vi "hardware_configurator.vi"() -> ()   [LabVIEW 2018]
doc: "MeasGUI - Measurement Graphics User Interface\nCopyright (c) 2018 Frans Korhonen\n\nMeasGUI was originally developed at Institute for Atmospheric \nand Earth System Research / Physics, Faculty of Science, \nUniversity of Helsinki, Finland\n\nAssistance, experience and feedback from following persons have been \ncritical in development of MeasGUI: Michel Attoui, Juha Kangasluoma, \nLauri Ahonen, Ella Häkkinen, Markku Kulmala and Tuukka Petäjä.\n\nThis file is part of MeasGUI.\n\nThis Source Code Form is subject to the terms of the Mozilla Public\nLicense, v. 2.0. If a copy of the MPL was not distributed with this\nfile, You can obtain one at http://mozilla.org/MPL/2.0/."
panel:
  in  "file cluster":T1={"open program folder"=FALSE, "Load"=FALSE, "Save"=FALSE, "Saved Configuration"="default", "output filename"="hardware.ini", "output"=FALSE}
  out "program path":path=path "C:/Users/fkorhone/projects/dmps_gui"
  out "saved controls":string[](array[string])=["NI measurement devices", "Serial ports"]
  in  "Tab Control":T2(tab)
  in  "NI measurement devices":T3(array[cluster])=[{"channel name"="NI1", "Device identifier"="Dev1", "analog outputs"=[{"channel name"="AO0", "terminal"="AO0"}, {"channel name"="AO1", "terminal"="AO1"}], "counter inputs"=[{"channel name"="counter", "resource"="ctr1", "terminal"="PFI0"}], "analog inputs"=[{"terminal"="AI0", "channel name"="AI0", "input terminal conf"="RSE", "signal min"=-10.0, "signal max"=10.0}, {"terminal"="AI1", "channel name"="AI1", "input terminal conf"="RSE", "signal min"=-10.0, "signal max"=10.0}], "pwm outputs"=[], "update period"=0.0, "sample rate"=0, "n average"=0}] {"update period" format="%.2f"}
  in  "Serial ports":T4(array[cluster])=[{"channel name"="serial1", "com port"="com10"}, {"channel name"="serial2", "com port"="com11"}, {"channel name"="serial3", "com port"="com12"}, {"channel name"="serial4", "com port"="com13"}]
  out "configuration":string="#CAUTION: Automatically generated file. Handmade modifications may be lost.\n\n#NI input device configuration:\ncreate niaidev NI1\ncreate timer NI1_period\nconf NI1_period 0.1\nconf NI1 Dev1 1000 10\n\n#Analog inputs:\ncreate niai AI0\nconf AI0 NI1 AI0 RSE -10.000000 10.000000\ncreate niai AI1\nconf AI1 NI1 AI1 RSE -10.000000 10.000000\n\nlink NI1_period NI1\n\n#Counter inputs:\ncreate nicounter counter\nsetup counter NI1 ctr1 PFI0\n\n#Analog outputs:\ncreate niao AO0\nsetup AO0 NI1 AO0\ncreate niao AO1\nsetup AO1 NI1 AO1\n\n#PWM outputs:\ncreate nipwm \nconf  0,000000 NI1  0\ncreate nipwm blower\nconf blower 1000,000000 NI1 ctr1 1\n\n#Serial configuration:\ncreate serial serial1 com10\ncreate serial serial2 com11\ncreate serial serial3 com12\ncreate serial serial4 com13\n"
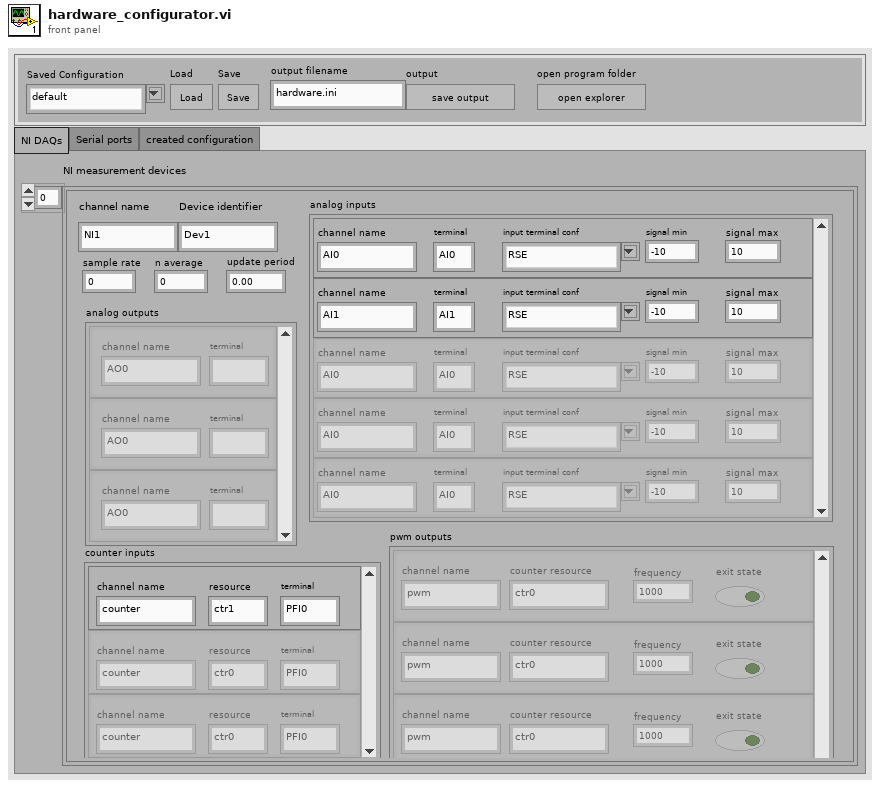
[diagram p1: front panel]
types:
  T1 = cluster{"open program folder":bool, "Load":bool, "Save":bool, "Saved Configuration":string, "output filename":string, "output":bool}
  T2 = enum32{"NI DAQs", "Serial ports", "created configuration"}
  T3 = cluster{"channel name":string, "Device identifier":string, "analog outputs":cluster{"channel name":string, "terminal":string}[], "counter inputs":cluster{"channel name":string, "resource":string, "terminal":string}[], "analog inputs":cluster{"terminal":string, "channel name":string, "input terminal conf":string, "signal min":dbl, "signal max":dbl}[], "pwm outputs":cluster{"channel name":string, "counter resource":string, "frequency":dbl, "exit state":bool}[], "update period":dbl, "sample rate":u32, "n average":u32}[]
  T4 = cluster{"channel name":string, "com port":string}[]
  T5 = enum16{"open", "replace", "create", "open or create", "replace or create", "replace or create with confirmation"}
  T6 = cluster{"channel name":string, "terminal":string}[]
  T7 = cluster{"channel name":string, "resource":string, "terminal":string}[]
  T8 = cluster{"terminal":string, "channel name":string, "input terminal conf":string, "signal min":dbl, "signal max":dbl}[]
  T9 = cluster{"channel name":string, "counter resource":string, "frequency":dbl, "exit state":bool}[]
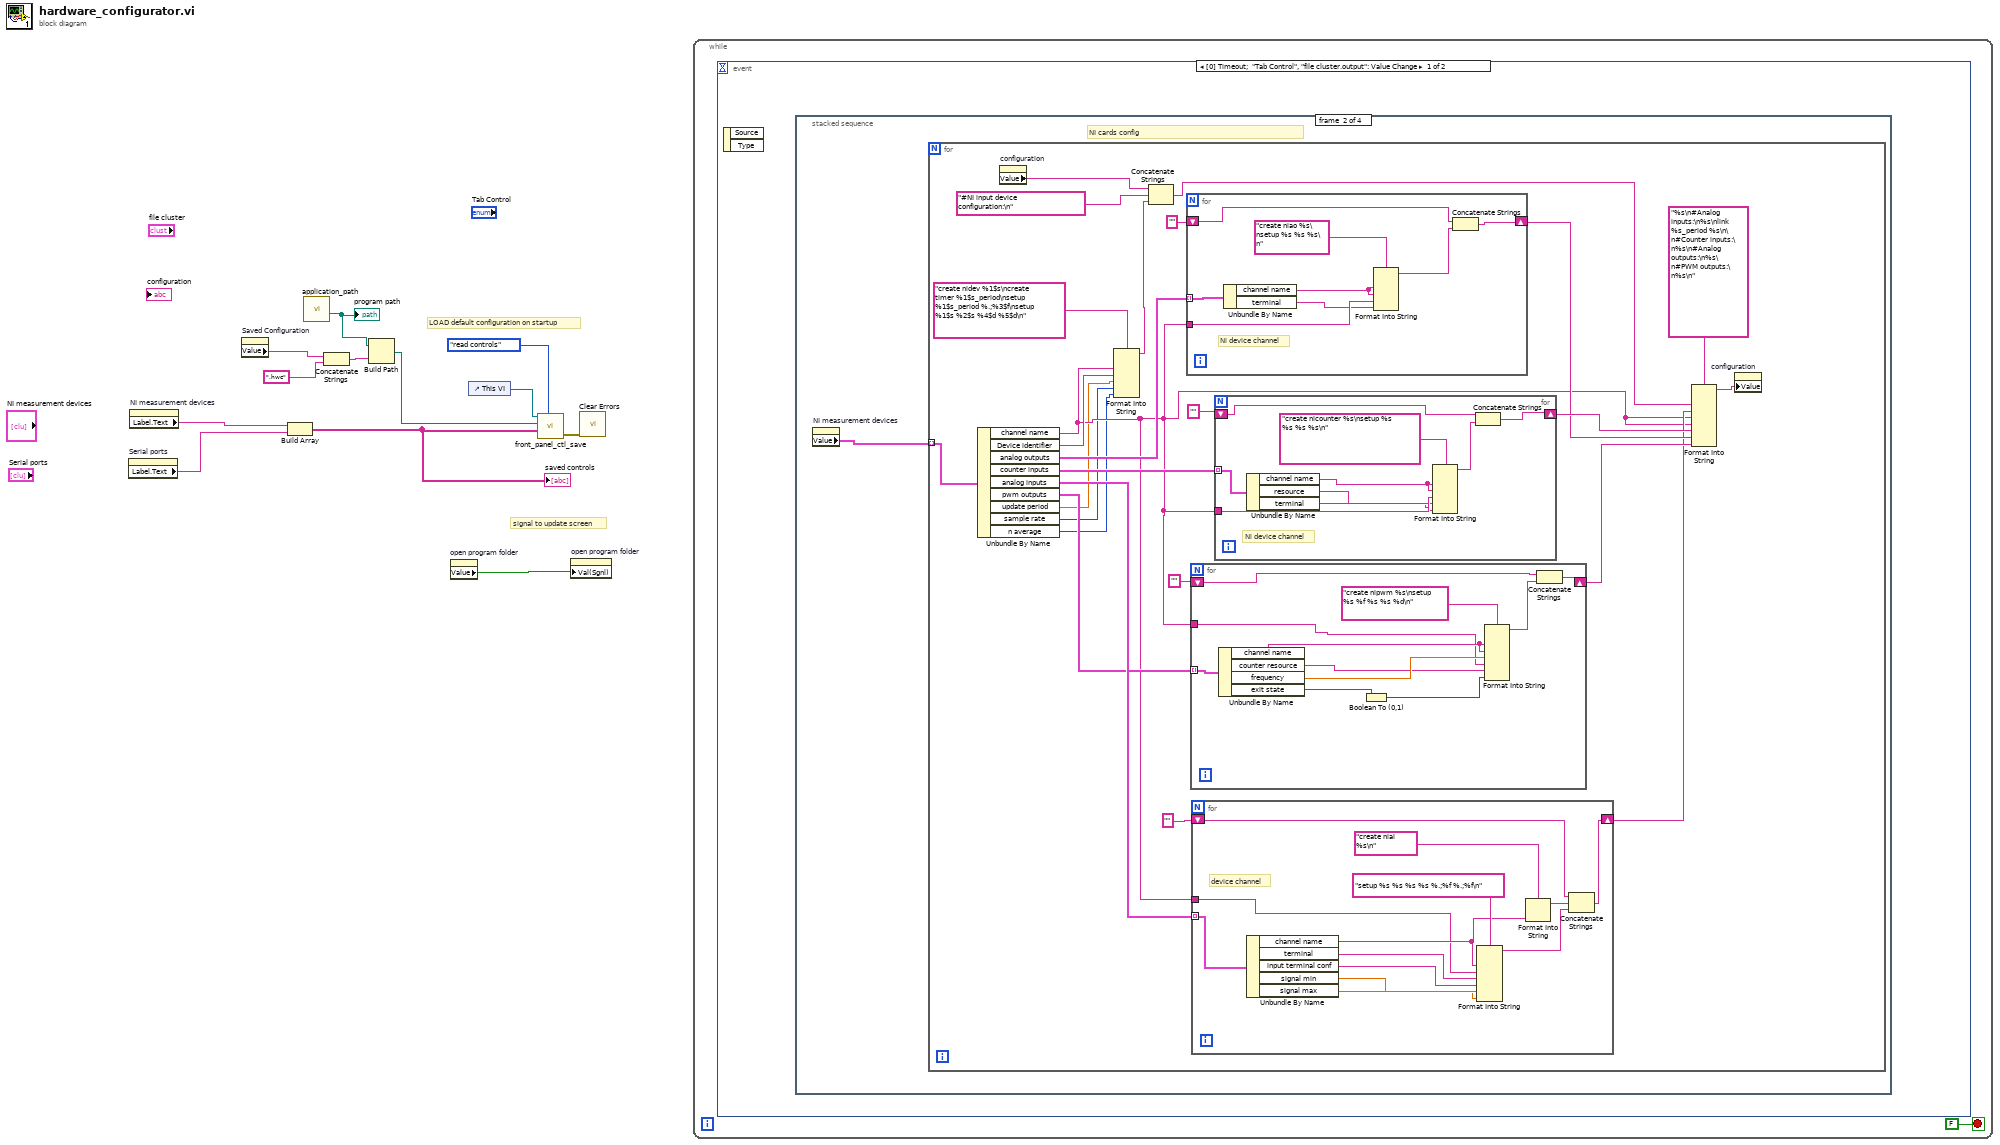
[diagram p0: block diagram]
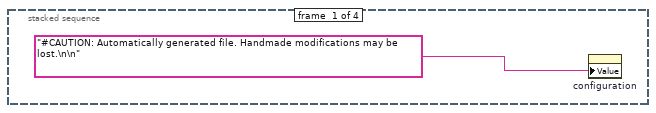
[diagram p2: hidden frame]
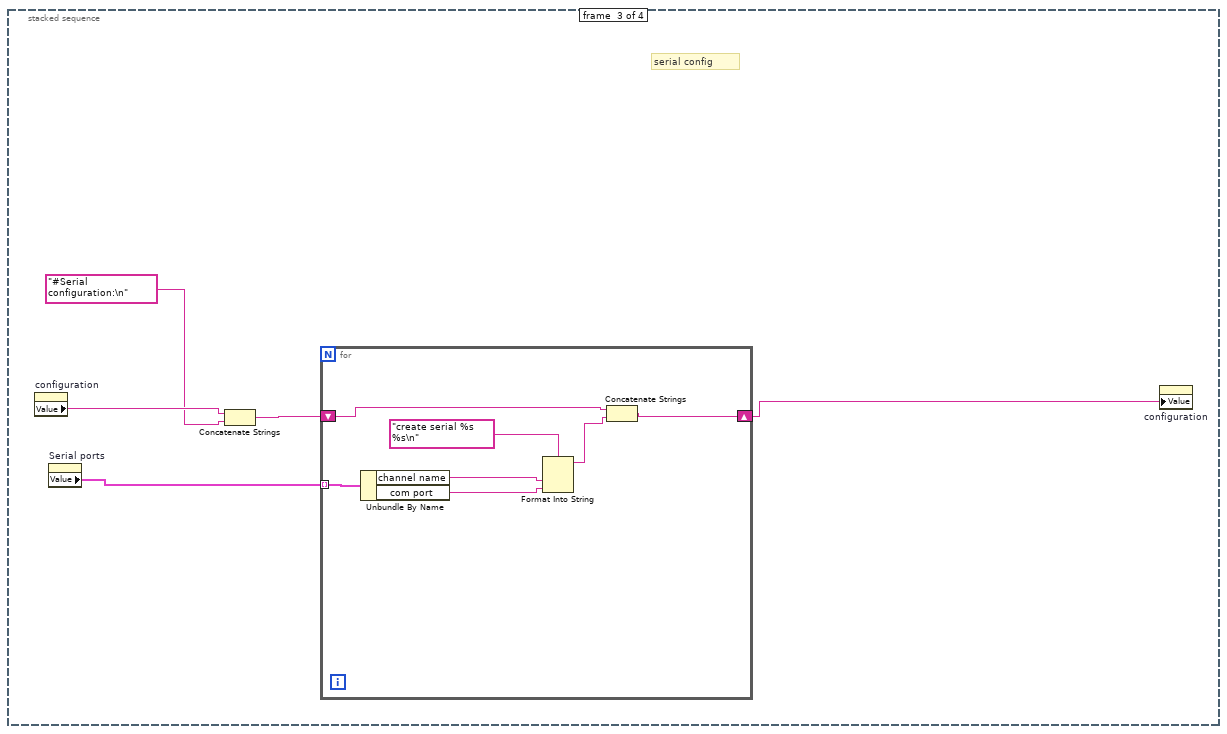
[diagram p3: hidden frame]
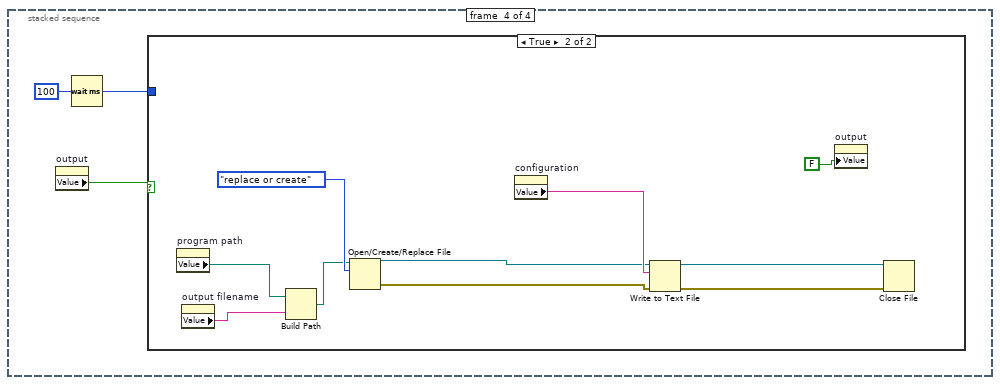
[diagram p4: hidden frame]
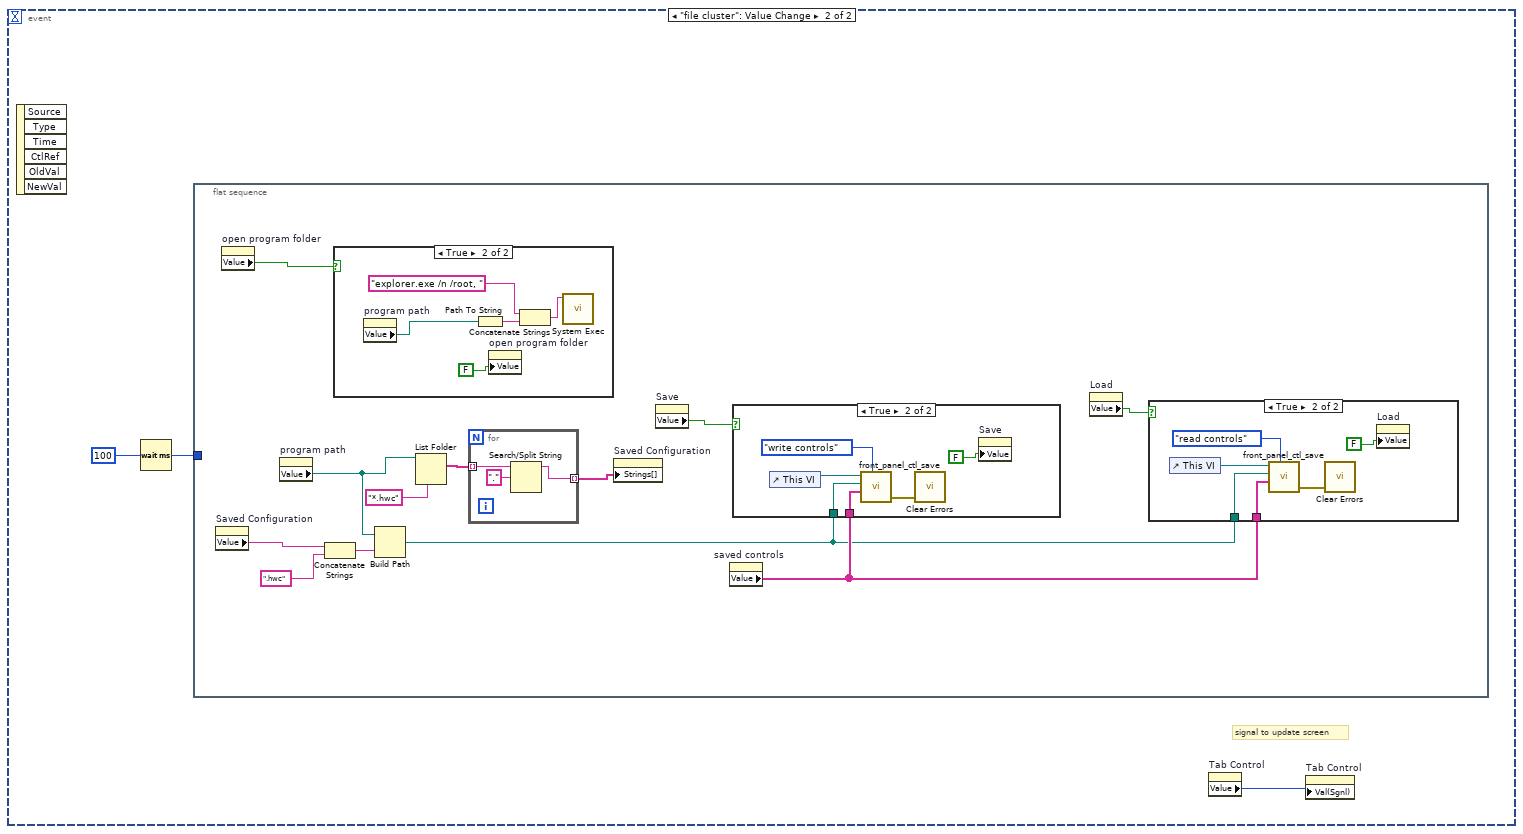
[diagram p6: hidden frame]
diagram:
  # "signal to update screen"
  # "LOAD default configuration on startup"
  n1 = property on="Serial ports" class="Arr (strict)"() -> ("Label.Text"=w3:string)  [unwired: 2 in, 2 out]
  n2 = property on="NI measurement devices" class="Arr (strict)"() -> ("Label.Text"=w4:string)  [unwired: 2 in, 2 out]
  n3 = property on="Saved Configuration" class="CmbBox"() -> ("Value"=w6:string)  [unwired: 2 in, 2 out]
  n4 = Build Array(w4, w3) -> (w5:string[])
  "saved controls" <- w5
  n5 = call "application_path.vi"() -> ("path"=w2:path)  [unwired: 11 in]
  "program path" <- w2
  n6 = Concatenate Strings(w6, ".hwc" ("string")) -> (w11:string)
  n7 = Build Path(base path=w2, name or relative path=w11) -> (appended path=w8:path)
  n8 = property on="open program folder" class="Bool (strict)"() -> ("Value"=w1:bool)  [unwired: 2 in, 2 out]
  n9 = control-ref of="This VI"() -> (w7:refnum<vi>)
  n10 = call "front_panel_ctl_save.vi"("VI in"=w7, "method"=enum16{"read controls", "write controls"}."read controls", "filename"=w8, "controls"=w5) -> ("error out"=w10:errorcluster)  [unwired: 4 in]
  n11 = property on="open program folder" class="Bool (strict)"("Val(Sgnl)"=w1) -> ()  [unwired: 2 in, 2 out]
  n12 = call <vilib>:"Clear Errors.vi"("error in (no error)"=w10) -> ()  [unwired: 5 in, 2 out]
  n13 = while {
    stop <- FALSE stop-if-true
    n14 = event shown="[0] Timeout;  \"Tab Control\", \"file cluster.output\": Value Change" {
      selector: _ -> [_ _]
      dyn-events: _ -> [_ _]
      timeout: _ -> [_ _]
      event Timeout; "Tab Control", "file cluster.output": Value Change {
        n15 = event-data() -> ()  [unwired: 1 in, 2 out]
        n16 = stacked-sequence {
          frame #0 {
            n17 = property on="configuration" class="Str"("Value"="#CAUTION: Automatically generated file. Handmade modifications may be lost.\n\n") -> ()  [unwired: 2 in, 2 out]
          }
          frame #1 {
            # "NI cards config"
            n18 = property on="NI measurement devices" class="Arr (strict)"() -> ("Value"=w15:T3)  [unwired: 2 in, 2 out]
            n19 = for {
              tunnel: w15 -> [w40] mode=indexing
              n20 = Unbundle By Name(w40) -> ("channel name"=w19:string, "Device identifier"=w20:string, "analog outputs"=w38:T6, "counter inputs"=w37:T7, "analog inputs"=w36:T8, "pwm outputs"=w26:T9, "update period"=w18:dbl, "sample rate"=w17:u32, "n average"=w16:u32)
              n21 = property on="configuration" class="Str"() -> ("Value"=w21:string)  [unwired: 2 in, 2 out]
              n22 = Format Into String(format string="create nidev %1$s\ncreate timer %1$s_period\nsetup %1$s_period %.;%3$f\nsetup %1$s %2$s %4$d %5$d\n", w19, w20, w18, w17, w16) -> (resulting string=w32:string)  [unwired: 2 in, 1 out]
              n23 = Concatenate Strings(w21, "#NI input device configuration:\n" ("string"), w32) -> (w23:string)
              n24 = for {
                tunnel: w38 -> [w81] mode=indexing
                tunnel: w19 -> [w78]
                shift-right: [w76] -> w28
                shift-left: "" -> [w75]
                # "Ni device channel"
                n25 = Unbundle By Name(w81) -> ("channel name"=w79:string, "terminal"=w77:string)
                n26 = Format Into String(format string="create niao %s\nsetup %s %s %s\n", w79, w79, w78, w77) -> (resulting string=w74:string)  [unwired: 2 in, 1 out]
                n27 = Concatenate Strings(w75, w74) -> (w76:string)
              }
              n28 = for {
                tunnel: w26 -> [w51] mode=indexing
                shift-right: [w48] -> w24
                shift-left: "" -> [w47]
                tunnel: w19 -> [w43]
                n29 = Unbundle By Name(w51) -> ("channel name"=w46:string, "counter resource"=w44:string, "frequency"=w45:dbl, "exit state"=w42:bool)
                n30 = Boolean To (0,1)(Boolean=w42) -> (0, 1=w41:i16)
                n31 = Format Into String(format string="create nipwm %s\nsetup %s %f %s %s %d\n", w46, w46, w45, w43, w44, w41) -> (resulting string=w49:string)  [unwired: 2 in, 1 out]
                n32 = Concatenate Strings(w47, w49) -> (w48:string)
              }
              n33 = for {
                tunnel: w36 -> [w64] mode=indexing
                tunnel: w19 -> [w60]
                shift-right: [w52] -> w22
                shift-left: "" -> [w53]
                # "device channel"
                n34 = Unbundle By Name(w64) -> ("channel name"=w61:string, "terminal"=w59:string, "input terminal conf"=w58:string, "signal min"=w57:dbl, "signal max"=w56:dbl)
                n35 = Format Into String(format string="setup %s %s %s %s %.;%f %.;%f\n", w61, w60, w59, w58, w57, w56) -> (resulting string=w54:string)  [unwired: 2 in, 1 out]
                n36 = Format Into String(format string="create niai %s\n", w61) -> (resulting string=w55:string)  [unwired: 2 in, 1 out]
                n37 = Concatenate Strings(w53, w55, w54) -> (w52:string)
              }
              n38 = for {
                tunnel: w37 -> [w73] mode=indexing
                tunnel: w19 -> [w67]
                shift-right: [w72] -> w30
                shift-left: "" -> [w71]
                # "Ni device channel"
                n39 = Unbundle By Name(w73) -> ("channel name"=w68:string, "resource"=w66:string, "terminal"=w65:string)
                n40 = Format Into String(format string="create nicounter %s\nsetup %s %s %s %s\n", w68, w68, w67, w66, w65) -> (resulting string=w69:string)  [unwired: 2 in, 1 out]
                n41 = Concatenate Strings(w71, w69) -> (w72:string)
              }
              n42 = Format Into String(format string="%s\n#Analog inputs:\n%s\nlink %s_period %s\n\n#Counter inputs:\n%s\n#Analog outputs:\n%s\n#PWM outputs:\n%s\n", w23, w22, w19, w19, w30, w28, w24) -> (resulting string=w29:string)  [unwired: 2 in, 1 out]
              n43 = property on="configuration" class="Str"("Value"=w29) -> ()  [unwired: 2 in, 2 out]
            }
          }
          frame #2 {
            # "serial config"
            n44 = property on="configuration" class="Str"() -> ("Value"=w85:string)  [unwired: 2 in, 2 out]
            n45 = property on="Serial ports" class="Arr (strict)"() -> ("Value"=w83:T4)  [unwired: 2 in, 2 out]
            n46 = Concatenate Strings(w85, "#Serial configuration:\n" ("format string")) -> (w86:string)
            n47 = for {
              tunnel: w83 -> [w93] mode=indexing
              shift-right: [w87] -> w82
              shift-left: w86 -> [w89]
              n48 = Unbundle By Name(w93) -> ("channel name"=w91:string, "com port"=w90:string)
              n49 = Format Into String(format string="create serial %s %s\n", w91, w90) -> (resulting string=w88:string)  [unwired: 2 in, 1 out]
              n50 = Concatenate Strings(w89, w88) -> (w87:string)
            }
            n51 = property on="configuration" class="Str"("Value"=w82) -> ()  [unwired: 2 in, 2 out]
          }
          frame #3 {
            n52 = property on="output" class="Bool (strict)"() -> ("Value"=w96:bool)  [unwired: 2 in, 2 out]
            n53 = Wait (ms)(milliseconds to wait=u32 100) -> (millisecond timer value=w94:u32)
            n54 = case shown="True" w96 {
              tunnel: w94 -> [_ _]
              frame False {
              }
              frame True {
                n55 = property on="program path" class="Path"() -> ("Value"=w98:path)  [unwired: 2 in, 2 out]
                n56 = property on="output filename" class="Str"() -> ("Value"=w99:string)  [unwired: 2 in, 2 out]
                n57 = Build Path(base path=w98, name or relative path=w99) -> (appended path=w97:path)
                n58 = Open/Create/Replace File(file path (use dialog)=w97, operation (0:open)=T5."replace or create") -> (refnum out=w101:refnum<file>, error out=w100:errorcluster)  [unwired: 4 in, 1 out]
                n59 = property on="configuration" class="Str"() -> ("Value"=w105:string)  [unwired: 2 in, 2 out]
                n60 = Write to Text File(file (use dialog)=w101, text=w105, error in=w100) -> (refnum out=w104:refnum<file>, error out=w103:errorcluster)  [unwired: 1 in, 1 out]
                n61 = property on="output" class="Bool (strict)"("Value"=FALSE) -> ()  [unwired: 2 in, 2 out]
                n62 = Close File(refnum=w104, error in=w103) -> ()  [unwired: 2 out]
              }
            }
          }
        }
      }
      event "file cluster": Value Change {
        # "signal to update screen"
        n63 = event-data() -> ()  [unwired: 1 in, 6 out]
        n64 = Wait (ms)(milliseconds to wait=u32 100) -> (millisecond timer value=w109:u32)
        n65 = flat-sequence {
          tunnel: w109 -> [_]
          frame #0 {
            n66 = property on="Saved Configuration" class="CmbBox"() -> ("Value"=w113:string)  [unwired: 2 in, 2 out]
            n67 = property on="open program folder" class="Bool (strict)"() -> ("Value"=w110:bool)  [unwired: 2 in, 2 out]
            n68 = property on="program path" class="Path"() -> ("Value"=w114:path)  [unwired: 2 in, 2 out]
            n69 = Concatenate Strings(w113, ".hwc" ("string")) -> (w119:string)
            n70 = case shown="True" w110 {
              frame False {
              }
              frame True {
                n71 = property on="program path" class="Path"() -> ("Value"=w123:path)  [unwired: 2 in, 2 out]
                n72 = Path To String(path=w123) -> (string=w124:string)
                n73 = property on="open program folder" class="Bool (strict)"("Value"=FALSE) -> ()  [unwired: 2 in, 2 out]
                n74 = Concatenate Strings("explorer.exe /n /root, " ("string"), w124) -> (w125:string)
                n75 = call <vilib>:"System Exec.vi"("command line"=w125) -> ()  [unwired: 7 in, 4 out]
              }
            }
            n76 = Build Path(base path=w114, name or relative path=w119) -> (appended path=w115:path)
            n77 = List Folder(path=w114, pattern="*.hwc") -> (filenames=w118:string[])  [unwired: 2 in, 3 out]
            n78 = for {
              tunnel: w118 -> [w129] mode=indexing
              tunnel: [w128] -> w117 mode=indexing
              n79 = Search/Split String(string=w129, search string/char (-)=".") -> (substring before match=w128:string)  [unwired: 1 in, 2 out]
            }
            n80 = property on="Saved Configuration" class="CmbBox"("Strings[]"=w117) -> ()  [unwired: 2 in, 2 out]
            n81 = property on="Save" class="Bool (strict)"() -> ("Value"=w111:bool)  [unwired: 2 in, 2 out]
            n82 = property on="saved controls" class="Arr (strict)"() -> ("Value"=w116:string[])  [unwired: 2 in, 2 out]
            n83 = case shown="True" w111 {
              tunnel: w116 -> [_ w139]
              tunnel: w115 -> [_ w138]
              frame False {
              }
              frame True {
                n84 = control-ref of="This VI"() -> (w141:refnum<vi>)
                n85 = call "front_panel_ctl_save.vi"("VI in"=w141, "method"=enum16{"read controls", "write controls"}."write controls", "filename"=w138, "controls"=w139) -> ("error out"=w136:errorcluster)  [unwired: 4 in]
                n86 = call <vilib>:"Clear Errors.vi"("error in (no error)"=w136) -> ()  [unwired: 5 in, 2 out]
                n87 = property on="Save" class="Bool (strict)"("Value"=FALSE) -> ()  [unwired: 2 in, 2 out]
              }
            }
            n88 = property on="Load" class="Bool (strict)"() -> ("Value"=w112:bool)  [unwired: 2 in, 2 out]
            n89 = case shown="True" w112 {
              tunnel: w116 -> [_ w132]
              tunnel: w115 -> [_ w133]
              frame False {
              }
              frame True {
                n90 = control-ref of="This VI"() -> (w134:refnum<vi>)
                n91 = call "front_panel_ctl_save.vi"("VI in"=w134, "method"=enum16{"read controls", "write controls"}."read controls", "filename"=w133, "controls"=w132) -> ("error out"=w130:errorcluster)  [unwired: 4 in]
                n92 = call <vilib>:"Clear Errors.vi"("error in (no error)"=w130) -> ()  [unwired: 5 in, 2 out]
                n93 = property on="Load" class="Bool (strict)"("Value"=FALSE) -> ()  [unwired: 2 in, 2 out]
              }
            }
          }
        }
        n94 = property on="Tab Control" class="TabCtl (strict)"() -> ("Value"=w107:T2)  [unwired: 2 in, 2 out]
        n95 = property on="Tab Control" class="TabCtl (strict)"("Val(Sgnl)"=w107) -> ()  [unwired: 2 in, 2 out]
      }
    }
  }
